vi "get_status.vi"(8 "error in (no error)":errorcluster, 11 "StageMH100301DMC in":refnum<class "StageMH100301DMC.lvclass">) -> (0 "error out":errorcluster, 2 "is happy?":bool=TRUE, 3 "StageMH100301DMC out":refnum<class "StageMH100301DMC.lvclass">)   [LabVIEW 2010, in "StageMH100301DMC.lvclass"]
uses:
  StageMH100301DMC.lvclass
  common/arrays/space_vector_array.ctl
  common/classes/SpaceVector/SpaceVector/SpaceVector.lvclass
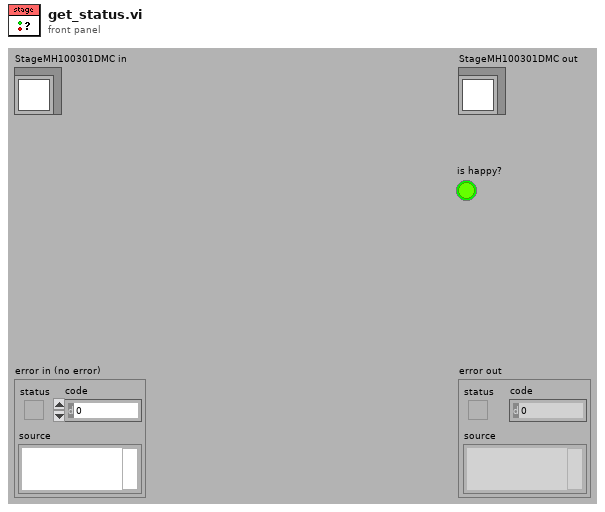
[diagram p1: front panel]
types:
  T1 = typedef "SpaceVector.lvclass/space_vector_array.ctl" = dbl[unit][]
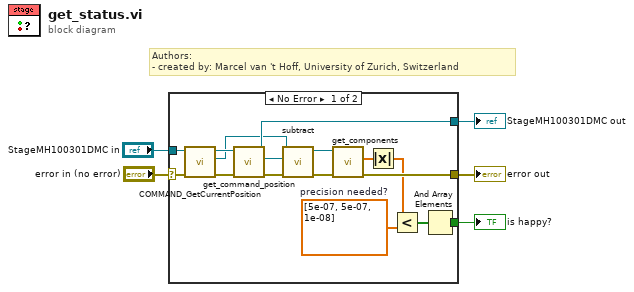
[diagram p0: block diagram]
diagram:
  # "Authors: \n- created by: Marcel van 't Hoff, University of Zurich, Switzerland"
  n1 = case shown="No Error" "error in (no error)" {
    selector: "error in (no error)" -> [w20 w22]
    tunnel: [w11 w22] -> w3
    tunnel: [w18 w23] -> w2
    tunnel: "StageMH100301DMC in" -> [w21 w23]
    tunnel: [w7 _] -> w1
    frame No Error {
      w10 = T1 [5e-07, 5e-07, 1e-08]  # precision needed?
      n2 = call-dynamic "COMMAND_GetCurrentPosition.vi"("error in (no error)"=w20, "MH100301DMC in"=w21) -> ("error out"=w17:errorcluster, "current position"=w16:refnum<class "SpaceVector.lvclass">, "MH100301DMC out"=w19:refnum<class "StageMH100301DMC.lvclass">)  [unwired: 7 in]
      n3 = call-dynamic "get_command_position.vi"("error in (no error)"=w17, "DL090409StageScaffold.lvclass in"=w19) -> ("error out"=w14:errorcluster, "SpaceVector.lvclass"=w15:refnum<class "SpaceVector.lvclass">, "DL090409StageScaffold.lvclass out"=w18:refnum<class "StageMH100301DMC.lvclass">)  [unwired: 7 out]
      n4 = call "subtract.vi"("error in (no error)"=w14, "subtrahend"=w15, "SpaceVector in"=w16) -> ("error out"=w12:errorcluster, "SpaceVector out"=w13:refnum<class "SpaceVector.lvclass">)  [unwired: 7 in]
      n5 = call "get_components.vi"("error in (no error)"=w12, "SpaceVector in"=w13) -> ("error out"=w11:errorcluster, "x/y/z"=w8:T1)  [unwired: 4 in, 4 out]
      n6 = Absolute Value(x=w8) -> (abs(x)=w6:T1)
      n7 = Less?(x=w6, y=w10) -> (x < y?=w9:bool[])
      n8 = And Array Elements(Boolean array=w9) -> (logical AND=w7:bool)
    }
    frame Error {
    }
  }
  "error out" <- w3
  "StageMH100301DMC out" <- w2
  "is happy?" <- w1
